vi "HumanDriveButtonBoxSourceClimb.vi"() -> ()   [LabVIEW 2023]
uses:
  <vilib>/Rock Robotics/WPI/ThirdParty/JAS_Junk/TrajLib/Trajectory_Library.lvlib
  HumanGlobal.vi
panel:
  out "DriveTraj":bool
  in  "Processor":bool
  in  "Climb":bool
  in  "LeftSourceLeft":bool
  in  "LeftSourceRight":bool
  in  "RightSourceLeft":bool
  in  "RightSourceRight":bool
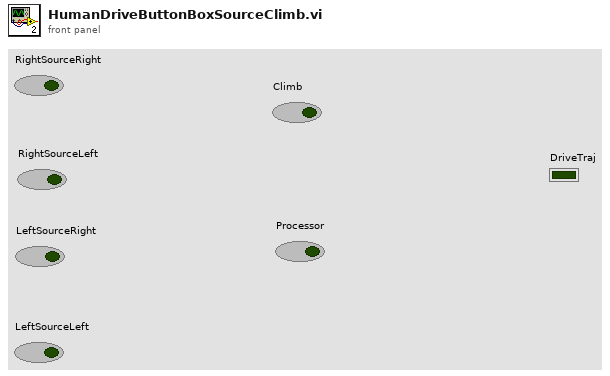
[diagram p1: front panel]
types:
  T1 = enum16{"NoTraj", "RightSourceRight", "RightSourceLeft", "LeftSourceRight", "LeftSourceLeft", "Climb", "Processor"}
  T2 = typedef "WPI_DriverStationAllianceInfo.ctl" = enum16{"Red", "Blue", "Invalid"}
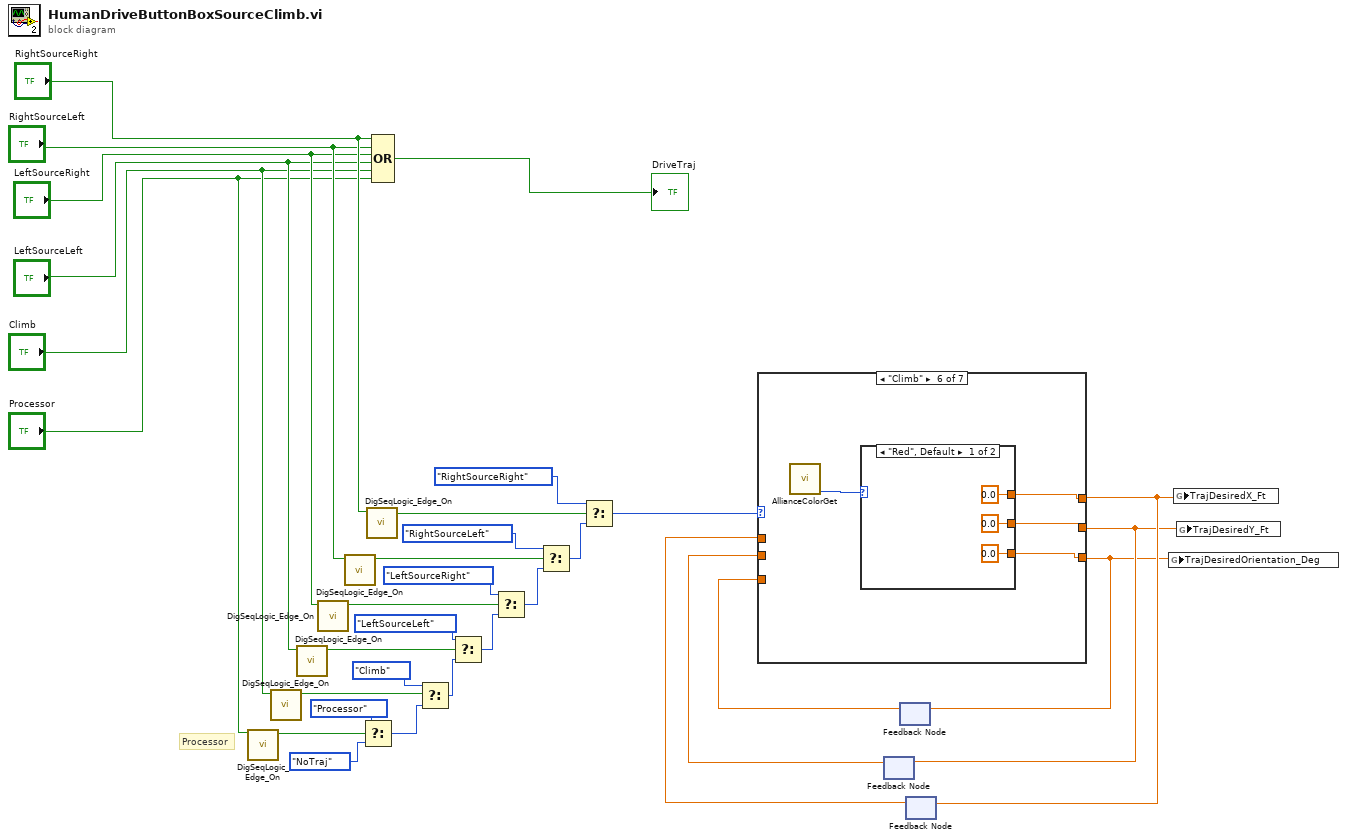
[diagram p0: block diagram]
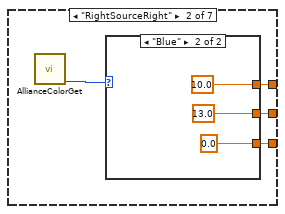
[diagram p3: hidden frame]
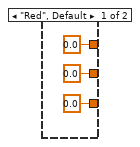
[diagram p4: hidden frame]
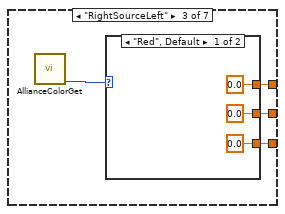
[diagram p5: hidden frame]
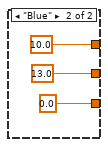
[diagram p6: hidden frame]
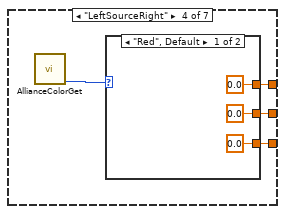
[diagram p7: hidden frame]
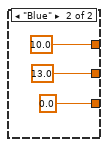
[diagram p8: hidden frame]
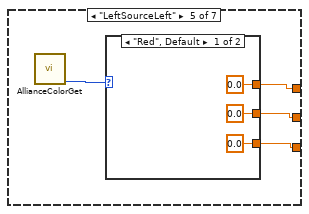
[diagram p9: hidden frame]
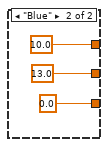
[diagram p10: hidden frame]
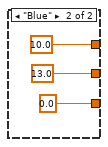
[diagram p11: hidden frame]
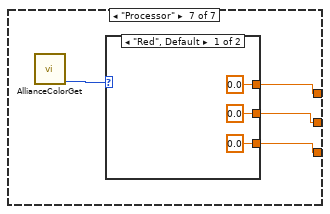
[diagram p12: hidden frame]
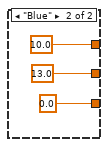
[diagram p13: hidden frame]
diagram:
  # "Processor"
  n1 = call <vilib>:"DigSeqLogic_Edge_On.vi"("Input"="Processor") -> ("On Edge"=w25:bool)  [unwired: 10 in]
  n2 = call <vilib>:"DigSeqLogic_Edge_On.vi"("Input"="Climb") -> ("On Edge"=w19:bool)  [unwired: 10 in]
  n3 = call <vilib>:"DigSeqLogic_Edge_On.vi"("Input"="LeftSourceLeft") -> ("On Edge"=w18:bool)  [unwired: 10 in]
  n4 = call <vilib>:"DigSeqLogic_Edge_On.vi"("Input"="LeftSourceRight") -> ("On Edge"=w17:bool)  [unwired: 10 in]
  n5 = call <vilib>:"DigSeqLogic_Edge_On.vi"("Input"="RightSourceLeft") -> ("On Edge"=w16:bool)  [unwired: 10 in]
  n6 = Select(t=T1."Processor", s=w25, f=T1."NoTraj") -> (s? t:f=w24:T1)
  n7 = call <vilib>:"DigSeqLogic_Edge_On.vi"("Input"="RightSourceRight") -> ("On Edge"=w15:bool)  [unwired: 10 in]
  n8 = Compound Arithmetic op=OR("RightSourceRight", "RightSourceLeft", "LeftSourceRight", "LeftSourceLeft", "Climb", "Processor") -> (→"DriveTraj":bool)
  n9 = Select(t=T1."Climb", s=w19, f=w24) -> (s? t:f=w23:T1)
  n10 = Select(t=T1."LeftSourceLeft", s=w18, f=w23) -> (s? t:f=w22:T1)
  n11 = Select(t=T1."LeftSourceRight", s=w17, f=w22) -> (s? t:f=w21:T1)
  n12 = Select(t=T1."RightSourceLeft", s=w16, f=w21) -> (s? t:f=w20:T1)
  n13 = Select(t=T1."RightSourceRight", s=w15, f=w20) -> (s? t:f=w7:T1)
  n14 = feedback #1() -> (w3:dbl)  [unwired: 1 in]
  n15 = feedback #2() -> (w1:dbl)  [unwired: 1 in]
  n16 = feedback #3() -> (w5:dbl)  [unwired: 1 in]
  n17 = case shown="\"Climb\"" w7 {
    tunnel: [w35 w39 w49 w59 w68 w78 w88] -> w6
    tunnel: [w34 w38 w48 w58 w67 w77 w87] -> w4
    tunnel: [w33 w37 w47 w57 w66 w76 w86] -> w2
    tunnel: w5 -> [w35 _ _ _ _ _ _]
    tunnel: w3 -> [w34 _ _ _ _ _ _]
    tunnel: w1 -> [w33 _ _ _ _ _ _]
    frame "NoTraj" {
    }
    frame "RightSourceRight" {
      n18 = call "AllianceColorGet.vi"() -> ("AllianceColor"=w36:T2)  [unwired: 11 in]
      n19 = case shown="\"Blue\"" w36 {
        tunnel: [0.0 ("TrajDesiredX_Ft") 10.0 ("TrajDesiredX_Ft")] -> w39
        tunnel: [0.0 ("TrajDesiredY_Ft") 13.0 ("TrajDesiredY_Ft")] -> w38
        tunnel: [0.0 ("TrajDesiredOrientation_Deg") 0.0 ("TrajDesiredOrientation_Deg")] -> w37
        frame "Red", Default {
        }
        frame "Blue" {
        }
      }
    }
    frame "RightSourceLeft" {
      n20 = call "AllianceColorGet.vi"() -> ("AllianceColor"=w46:T2)  [unwired: 11 in]
      n21 = case shown="\"Red\", Default" w46 {
        tunnel: [0.0 ("TrajDesiredX_Ft") 10.0 ("TrajDesiredX_Ft")] -> w49
        tunnel: [0.0 ("TrajDesiredY_Ft") 13.0 ("TrajDesiredY_Ft")] -> w48
        tunnel: [0.0 ("TrajDesiredOrientation_Deg") 0.0 ("TrajDesiredOrientation_Deg")] -> w47
        frame "Red", Default {
        }
        frame "Blue" {
        }
      }
    }
    frame "LeftSourceRight" {
      n22 = call "AllianceColorGet.vi"() -> ("AllianceColor"=w56:T2)  [unwired: 11 in]
      n23 = case shown="\"Red\", Default" w56 {
        tunnel: [0.0 ("TrajDesiredX_Ft") 10.0 ("TrajDesiredX_Ft")] -> w59
        tunnel: [0.0 ("TrajDesiredY_Ft") 13.0 ("TrajDesiredY_Ft")] -> w58
        tunnel: [0.0 ("TrajDesiredOrientation_Deg") 0.0 ("TrajDesiredOrientation_Deg")] -> w57
        frame "Red", Default {
        }
        frame "Blue" {
        }
      }
    }
    frame "LeftSourceLeft" {
      n24 = call "AllianceColorGet.vi"() -> ("AllianceColor"=w69:T2)  [unwired: 11 in]
      n25 = case shown="\"Red\", Default" w69 {
        tunnel: [0.0 ("TrajDesiredX_Ft") 10.0 ("TrajDesiredX_Ft")] -> w68
        tunnel: [0.0 ("TrajDesiredY_Ft") 13.0 ("TrajDesiredY_Ft")] -> w67
        tunnel: [0.0 ("TrajDesiredOrientation_Deg") 0.0 ("TrajDesiredOrientation_Deg")] -> w66
        frame "Red", Default {
        }
        frame "Blue" {
        }
      }
    }
    frame "Climb" {
      n26 = call "AllianceColorGet.vi"() -> ("AllianceColor"=w79:T2)  [unwired: 11 in]
      n27 = case shown="\"Red\", Default" w79 {
        tunnel: [0.0 ("TrajDesiredX_Ft") 10.0 ("TrajDesiredX_Ft")] -> w78
        tunnel: [0.0 ("TrajDesiredY_Ft") 13.0 ("TrajDesiredY_Ft")] -> w77
        tunnel: [0.0 ("TrajDesiredOrientation_Deg") 0.0 ("TrajDesiredOrientation_Deg")] -> w76
        frame "Red", Default {
        }
        frame "Blue" {
        }
      }
    }
    frame "Processor" {
      n28 = call "AllianceColorGet.vi"() -> ("AllianceColor"=w89:T2)  [unwired: 11 in]
      n29 = case shown="\"Red\", Default" w89 {
        tunnel: [0.0 ("TrajDesiredX_Ft") 10.0 ("TrajDesiredX_Ft")] -> w88
        tunnel: [0.0 ("TrajDesiredY_Ft") 13.0 ("TrajDesiredY_Ft")] -> w87
        tunnel: [0.0 ("TrajDesiredOrientation_Deg") 0.0 ("TrajDesiredOrientation_Deg")] -> w86
        frame "Red", Default {
        }
        frame "Blue" {
        }
      }
    }
  }
  n30 = feedback-in #1(w4) -> ()
  n31 = feedback-in #2(w2) -> ()
  n32 = feedback-in #3(w6) -> ()
  n33 = global write "HumanGlobal.vi" "TrajDesiredOrientation_Deg"(w2) -> ()
  n34 = global write "HumanGlobal.vi" "TrajDesiredX_Ft"(w6) -> ()
  n35 = global write "HumanGlobal.vi" "TrajDesiredY_Ft"(w4) -> ()
